vi "HK Read Channels.vi"(11 "Channel Name":string) -> (1 "Std. Dev.":dbl, 2 "Running Avg.":dbl, 3 "Value":dbl)   [LabVIEW 2024, in "HK Table.lvclass"]
uses:
  HK Table.lvclass
  RIMAS/Logging/CC enum Current Values Action.ctl
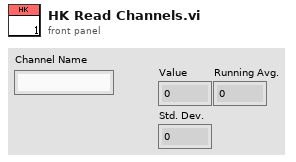
[diagram p1: front panel]
types:
  T1 = typedef "CC enum Current Values Action.ctl" = enum16{"Init", "Write Item", "Write Array", "Read Item", "Read Array", "Read All", "Add Channels", "New File", "Add Message", "Get Current Values", "Close"}
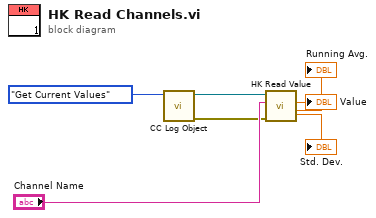
[diagram p0: block diagram]
diagram:
  n1 = call "CC Log Object.vi"("Action"=CC_enum_Current_Values_Action."Get Current Values") -> ("error out"=w4:errorcluster, "HK Channel out"=w6:refnum<class "HK Table.lvclass">)  [unwired: 8 in, 1 out]
  n2 = call-dynamic "HK Read Value.vi"("error in (no error)"=w4, "Channel Name"="Channel Name", "HK Channel in"=w6) -> ("Running Avg."=→"Running Avg.":dbl, "Value"=→"Value":dbl, "Std. Dev."=→"Std. Dev.":dbl)  [unwired: 3 in, 3 out]
